vi "Hella CAN.vi"(8 "Error IN":errorcluster, 10 "Re-Init CAN":bool, 11 "CMD":u8) -> (0 "Error OUT":errorcluster)   [LabVIEW 2019]
uses:
  Type Defs/CAN Mode.ctl
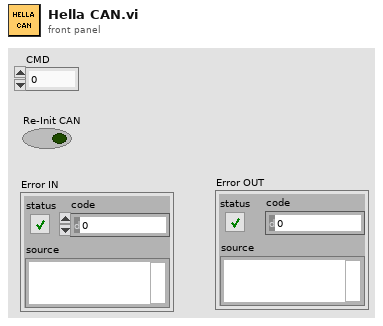
[diagram p1: front panel]
types:
  T1 = typedef "CAN Mode.ctl" = enum16{"Init", "Read", "Write", "Close"}
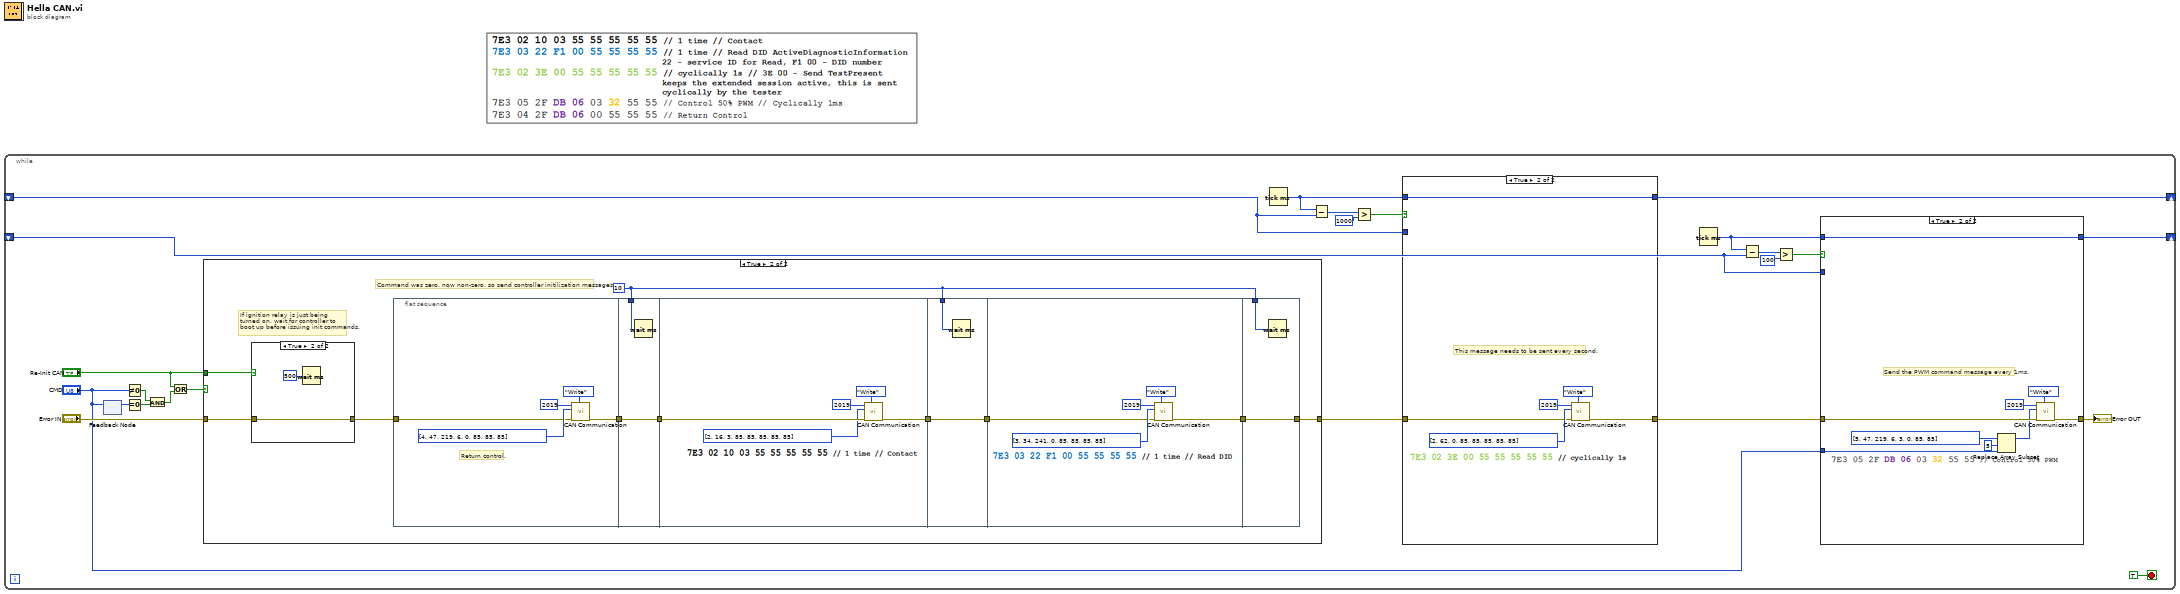
[diagram p0: block diagram]
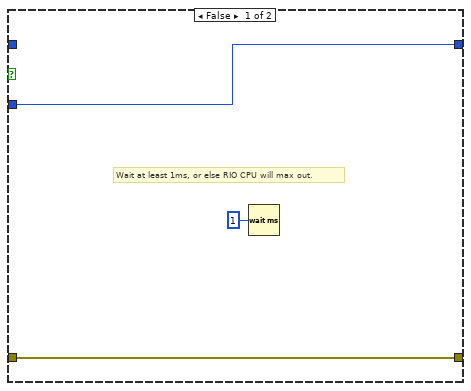
[diagram p2: hidden frame]
diagram:
  n1 = while {
    shift-right: [w21] -> _
    shift-left: _ -> [w20]
    shift-right: [w19] -> _
    shift-left: _ -> [w18]
    stop <- TRUE stop-if-true
    n2 = feedback #1() -> (w24:u8)  [unwired: 1 in]
    n3 = feedback-in #1("CMD") -> ()
    n4 = Not Equal To 0?(x="CMD") -> (x != 0?=w4:bool)
    n5 = Equal To 0?(x=w24) -> (x = 0?=w6:bool)
    n6 = And(x=w4, y=w6) -> (x .and. y?=w3:bool)
    n7 = Or(x="Re-Init CAN", y=w3) -> (x .or. y?=w1:bool)
    n8 = case shown="True" w1 {
      tunnel: "Error IN" -> [w45 w53]
      tunnel: [w45 w55] -> w17
      tunnel: "Re-Init CAN" -> [_ w54]
      frame False {
        # "Should have communication with the controller, so don't send initilization messages."
      }
      frame True {
        w46 = u32 10 ("milliseconds to wait")
        # "Command was zero, now non-zero, so send controller initilization messages."
        # "If ignition relay is just being\nturned on, wait for controller to\nboot up before issuing init commands."
        n9 = case shown="True" w54 {
          tunnel: [w77 w78] -> w52
          tunnel: w53 -> [w77 w78]
          frame False {
          }
          frame True {
            n10 = Wait (ms)(milliseconds to wait=u32 500) -> ()  [unwired: 1 out]
          }
        }
        n11 = flat-sequence {
          tunnel: [w58] -> w51
          tunnel: w52 -> [w56]
          tunnel: w51 -> [w62]
          tunnel: [w62] -> w50
          tunnel: w46 -> [w61]
          tunnel: [w67] -> w49
          tunnel: w50 -> [w66]
          tunnel: w46 -> [w69]
          tunnel: [w68] -> w48
          tunnel: w49 -> [w68]
          tunnel: w48 -> [w71]
          tunnel: [w70] -> w47
          tunnel: w46 -> [w76]
          tunnel: w47 -> [w75]
          tunnel: [w75] -> w55
          frame #0 {
            # "Return control."
            n12 = call "CAN Communication.vi"("CAN Mode"=CAN_Mode."Write", "Error IN"=w56, "Message"=u8[] [4, 47, 219, 6, 0, 85, 85, 85] ("array"), "Arbitration ID"=u32 2019 ("CAN Addres to Xmit\nSpeed CMD (Hex) 2")) -> ("Error OUT"=w58:errorcluster)  [unwired: 6 in, 1 out]
          }
          frame #1 {
            n13 = Wait (ms)(milliseconds to wait=w61) -> ()  [unwired: 1 out]
          }
          frame #2 {
            n14 = call "CAN Communication.vi"("CAN Mode"=CAN_Mode."Write", "Error IN"=w66, "Message"=u8[] [2, 16, 3, 85, 85, 85, 85, 85] ("array"), "Arbitration ID"=u32 2019 ("CAN Addres to Xmit\nSpeed CMD (Hex) 2")) -> ("Error OUT"=w67:errorcluster)  [unwired: 6 in, 1 out]
          }
          frame #3 {
            n15 = Wait (ms)(milliseconds to wait=w69) -> ()  [unwired: 1 out]
          }
          frame #4 {
            n16 = call "CAN Communication.vi"("CAN Mode"=CAN_Mode."Write", "Error IN"=w71, "Message"=u8[] [3, 34, 241, 0, 85, 85, 85, 85] ("array"), "Arbitration ID"=u32 2019 ("CAN Addres to Xmit\nSpeed CMD (Hex) 2")) -> ("Error OUT"=w70:errorcluster)  [unwired: 6 in, 1 out]
          }
          frame #5 {
            n17 = Wait (ms)(milliseconds to wait=w76) -> ()  [unwired: 1 out]
          }
        }
      }
    }
    n18 = Tick Count (ms)() -> (millisecond timer value=w14:u32)
    n19 = Subtract(x=w14, y=w20) -> (x-y=w16:u32)
    n20 = Greater?(x=w16, y=u32 1000) -> (0:w8:bool)
    n21 = case shown="True" w8 {
      tunnel: w17 -> [w37 w41]
      tunnel: [w38 w40] -> w21
      tunnel: w14 -> [_ w40]
      tunnel: w20 -> [w38 _]
      tunnel: [w37 w39] -> w10
      frame False {
      }
      frame True {
        # "This message needs to be sent every second."
        n22 = call "CAN Communication.vi"("CAN Mode"=CAN_Mode."Write", "Error IN"=w41, "Message"=u8[] [2, 62, 0, 85, 85, 85, 85, 85] ("array"), "Arbitration ID"=u32 2019 ("CAN Addres to Xmit\nSpeed CMD (Hex) 2")) -> ("Error OUT"=w39:errorcluster)  [unwired: 6 in, 1 out]
      }
    }
    n23 = Tick Count (ms)() -> (millisecond timer value=w11:u32)
    n24 = Subtract(x=w11, y=w18) -> (x-y=w12:u32)
    n25 = Greater?(x=w12, y=u32 100) -> (0:w7:bool)
    n26 = case shown="True" w7 {
      tunnel: w10 -> [w26 w34]
      tunnel: [w27 w33] -> w19
      tunnel: w11 -> [_ w33]
      tunnel: w18 -> [w27 _]
      tunnel: "CMD" -> [_ w28]
      tunnel: [w26 w29] -> w9
      frame False {
        # "Wait at least 1ms, or else RIO CPU will max out."
        n27 = Wait (ms)(milliseconds to wait=u32 1) -> ()  [unwired: 1 out]
      }
      frame True {
        # "Send the PWM command message every 1ms."
        n28 = Replace Array Subset(array=u8[] [5, 47, 219, 6, 3, 0, 85, 85], new element=w28, index=5) -> (w30:u8[])
        n29 = call "CAN Communication.vi"("CAN Mode"=CAN_Mode."Write", "Error IN"=w34, "Message"=w30, "Arbitration ID"=u32 2019 ("CAN Addres to Xmit\nSpeed CMD (Hex) 2")) -> ("Error OUT"=w29:errorcluster)  [unwired: 6 in, 1 out]
      }
    }
    "Error OUT" <- w9
  }
